vi "Arm Controller.vi"(8 "error in":errorcluster) -> ()   [LabVIEW 2018]
doc: "This VI executes continuously carrying out the current operation and responding to updates or new operations. It will often contain the timing or control code that is difficult to place directly in TeleOp. This VI generally opens all sensors and motors and isolates the rest of the robot code from knowing how the operations are carried out."
uses:
  <vilib>/Rock Robotics/WPI/Framework/Completion Status.ctl
  Arm Setpoints.ctl
  Arm Operations.ctl
  <vilib>/Rock Robotics/SystemInterfaces/AI/FPGA_AIChannel.ctl
  <vilib>/Rock Robotics/WPI/SafetyOutput/WPI_SafetyOutputConfigMenu.ctl
  <vilib>/Rock Robotics/SystemInterfaces/DIO/FPGA_DIOPWMChannel.ctl
  <vilib>/Rock Robotics/WPI/MotorControl/WPI_MotorControlOpen SPARK.vi
panel:
  in  "g":dbl=0.15 format="%#_13g"
  out "POT Angle":dbl
  in  "output range":cluster{"output high":dbl, "output low":dbl}={"output high"=1.0, "output low"=-0.75} {"output low" format="%.2f"; "output high" format="%.2f"}
  in  "PIDF gains":cluster{"Kp":dbl, "Ki":dbl, "Kd":dbl, "Kf":dbl}={"Kp"=0.08, "Ki"=0.0, "Kd"=0.05, "Kf"=0.0} {"Kf" format="%.3f"; "Kd" format="%.3f"; "Ki" format="%.3f"; "Kp" format="%.3f"}
  out "MotorPower":dbl(graph)
  in  "0 voltage":dbl(slide)=2.93 min=0.0 max=5.0 scale=0.0..5.0
  out "POT Voltage":dbl
  out "POT":cluster{"Normalized Value":dbl, "Setpoint":dbl}(graph)
  in  "Max angle":dbl=80.0
  in  "Min angle":dbl=-85.0
  in  "Interactive Values":T1
  out "Current\nCmd":string
  in  "Buttons":cluster{"Execute Cmd":bool, "Abort Cmd":bool}
  out "Command Timing":cluster{"Start Time (ms)":u32, "Iterations":i32}
  out "Status":T3
  # "Interactive Command: You may fill in the settings for a command\nand schedule it with the Execute button. You can observe and abort\nany command while fine tuning the code for the controller."
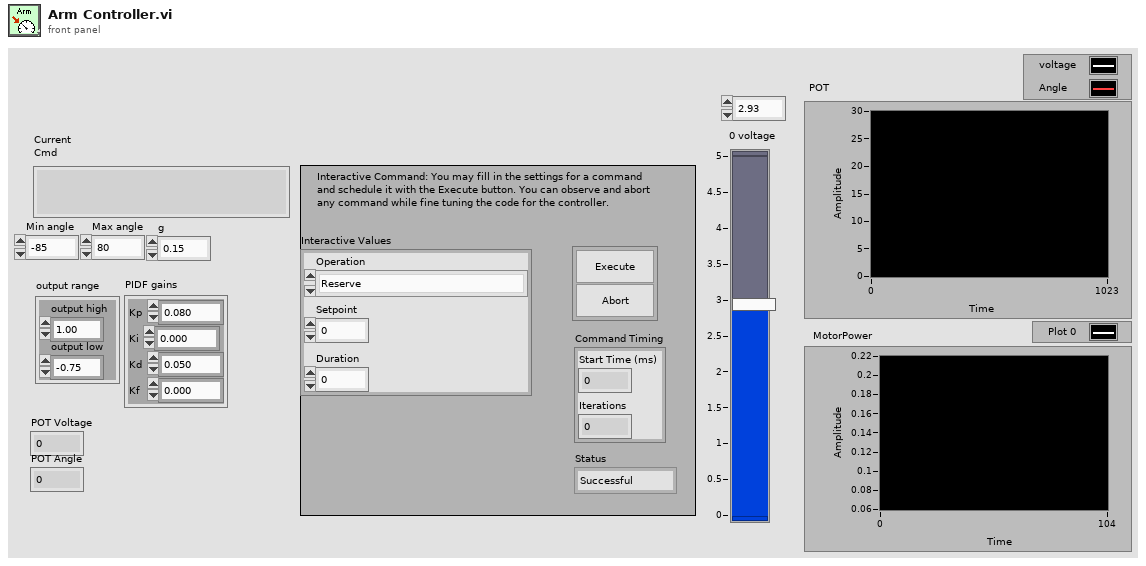
[diagram p1: front panel]
types:
  T1 = typedef "Arm Setpoints.ctl" = cluster{"Operation":T2, "Setpoint":dbl, "Duration":dbl}
  T2 = typedef "Arm Operations.ctl" = enum16{"Reserve", "Read Current", "Turn to angle ", "Set position", "Immediate"}
  T3 = typedef "Completion Status.ctl" = enum16{"Successful", "Aborted", "Incomplete"}
  T4 = typedef "FPGA_DIOPWMChannel.ctl" = enum8{"PWM 0", "PWM 1", "PWM 2", "PWM 3", "PWM 4", "PWM 5", "PWM 6", "PWM 7", "PWM 8", "PWM 9", "PWM MXP 0", "PWM MXP 1", "PWM MXP 2", "PWM MXP 3", "PWM MXP 4", "PWM MXP 5", "PWM MXP 6", "PWM MXP 7", "PWM MXP 8", "PWM MXP 9", "Invalid"}
  T5 = typedef "WPI_SafetyOutputConfigMenu.ctl" = enum16{"Enable", "Disable"}
  T6 = typedef "FPGA_AIChannel.ctl" = enum8{"AI 0", "AI 1", "AI 2", "AI 3", "AI MXP 0", "AI MXP 1", "AI MXP 2", "AI MXP 3", "Invalid"}
  T7 = typedef "WPI_AnalogChannelDevRef.ctl" = cluster{"DevStatus":errorcluster, "Analog Channel":T6}
  T8 = typedef "WPI_MotorControlDeviceRef.ctl" = cluster{"DeviceStatus":errorcluster, "Type":T9, "PWM":cluster{"PWM Channel":T4, "DeadBand":T10}, "CAN":cluster{"Device Number":u8, "SetOutput VI Ref":variant, "GetOutput VI Ref":variant, "Enable VI Ref":variant, "Disable VI Ref":variant, "Data":variant}, "Invert":bool, "DIO PWM":cluster{"PWM \"Enable\" Channel":T4, "DIOChannel":T11, "PWM Rate":dbl}}
  T9 = typedef "WPI_MotorControlType.ctl" = enum16{"PWM", "CAN", "DIO PWM"}
  T10 = typedef "WPI_PWMDeadband.ctl" = cluster{"Name":string, "maxPositivePwm":i32, "minPositivePwm":i32, "centerPwm":i32, "maxNegativePwm":i32, "minNegativePwm":i32, "angularRange":u16}
  T11 = typedef "FPGA_DIOChannel.ctl" = enum8{"DIO 0", "DIO 1", "DIO 2", "DIO 3", "DIO 4", "DIO 5", "DIO 6", "DIO 7", "DIO 8", "DIO 9", "DIO MXP 0", "DIO MXP 1", "DIO MXP 2", "DIO MXP 3", "DIO MXP 4", "DIO MXP 5", "DIO MXP 6", "DIO MXP 7", "DIO MXP 8", "DIO MXP 9", "DIO MXP 10", "DIO MXP 11", "DIO MXP 12", "DIO MXP 13", "DIO MXP 14", "DIO MXP 15", "SPI Port CS1", "SPI Port CS2", "SPI Port CS3", "SPI Port MISO", "SPI Port MOSI", "Invalid"}
  T12 = typedef "Command Status Info.ctl" = cluster{"Name":string, "Status":T3, "notifier out":T13}
  T13 = typedef "Completion Notifier.ctl" = refnum<notifier>
  T14 = cluster{"Current Command":T1, "Command Timing":cluster{"Start Time (ms)":u32, "Iterations":i32}, "Command Arguments":cluster{"Command Info":T12, "Description":string, "Default Command":T1, "queue out":refnum<queue>, "Subsystem Name":string}}
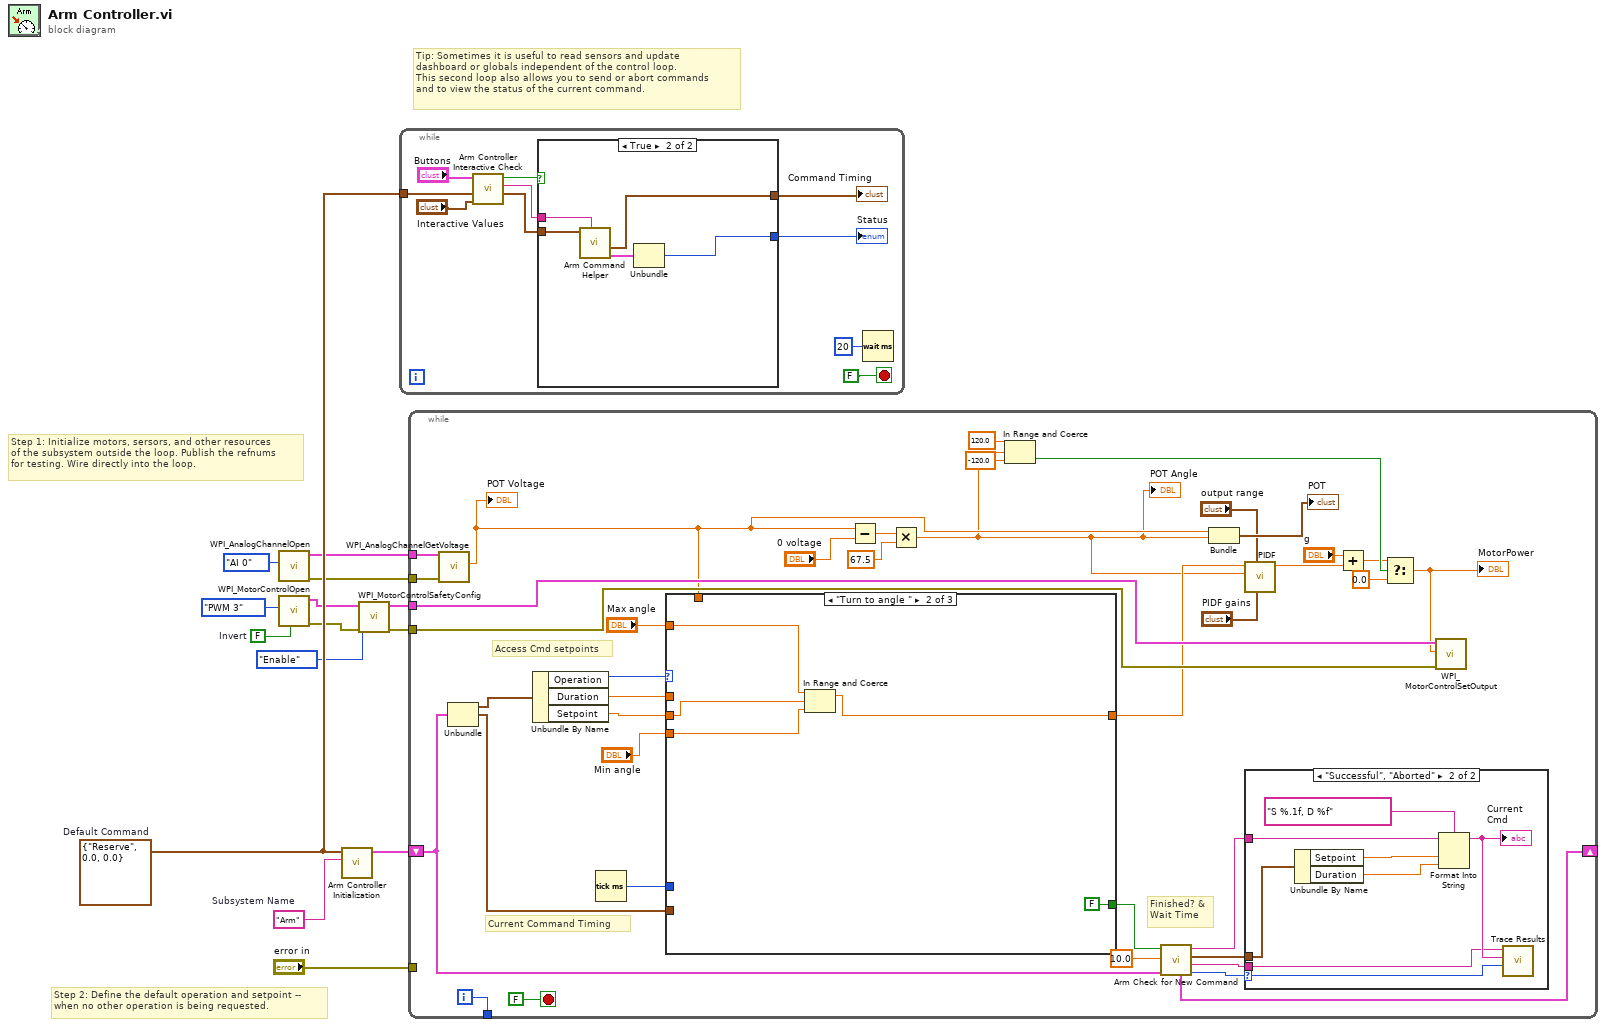
[diagram p0: block diagram]
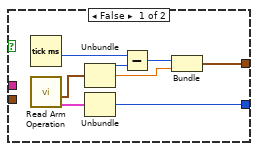
[diagram p2: hidden frame]
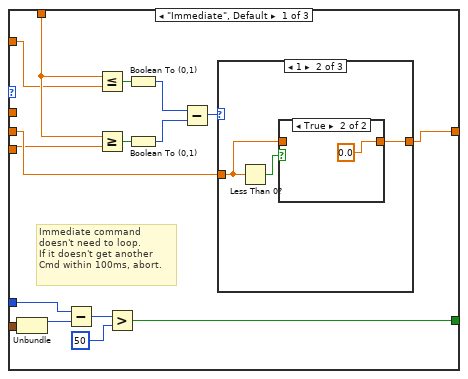
[diagram p4: hidden frame]
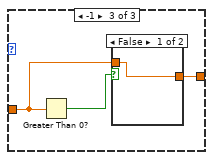
[diagram p7: hidden frame]
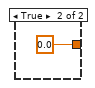
[diagram p8: hidden frame]
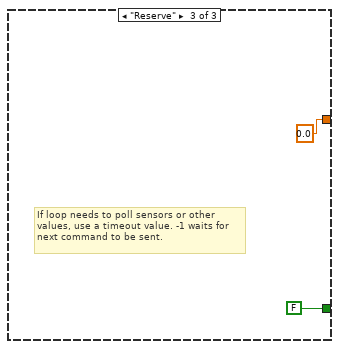
[diagram p9: hidden frame]
diagram:
  w1 = FALSE  # Invert
  w11 = T1 {"Operation"=enum."Reserve", "Setpoint"=0.0, "Duration"=0.0}  # Default Command
  w12 = "Arm"  # Subsystem Name
  # "Tip: Sometimes it is useful to read sensors and update\ndashboard or globals independent of the control loop.\nThis second loop also allows you to send or abort commands\nand to view the status of the current command."
  # "Step 2: Define the default operation and setpoint --\nwhen no other operation is being requested."
  # "Step 1: Initialize motors, sersors, and other resources\nof the subsystem outside the loop. Publish the refnums\nfor testing. Wire directly into the loop."
  n1 = call <vilib>:"WPI_AnalogChannelOpen.vi"("Analog Channel"=FPGA_AIChannel."AI 0") -> ("error out"=w10:errorcluster, "AIDeviceRef"=w9:T7)  [unwired: 9 in]
  n2 = call-poly <vilib>:"WPI_MotorControlOpen.vi"("Invert"=w1, "PWM Channel"=FPGA_DIOPWMChannel."PWM 3") -> ("error out"=w6:errorcluster, "MotorControlDeviceRef"=w7:T8)  [unwired: 8 in]
  n3 = call "Arm Controller Initialization.vi"("Subsystem Name"=w12, "Default Command"=w11) -> ("Current Command"=w13:T14)  [unwired: 9 in]
  n4 = call <vilib>:"WPI_MotorControlSafetyConfig.vi"("error in (no error)"=w6, "mode"=WPI_SafetyOutputConfigMenu."Enable", "MotorControlDevRef"=w7) -> ("error out"=w4:errorcluster, "MotorControlDevRef"=w5:T8)  [unwired: 7 in]
  n5 = while {
    tunnel: w11 -> [w21]
    stop <- FALSE stop-if-true
    n6 = call "Arm Controller Interactive Check.vi"("Interactive Command in"="Interactive Values", "Default Command"=w21, "Buttons"="Buttons") -> ("Interactive Command out"=w18:T1, "Trace String"=w19:string, "Schedule"=w20:bool)  [unwired: 6 in]
    n7 = case shown="True" w20 {
      tunnel: [w32 w37] -> w17
      tunnel: w18 -> [_ w35]
      tunnel: [w28 w33] -> w16
      tunnel: w19 -> [_ w36]
      frame False {
        n8 = Tick Count (ms)() -> (millisecond timer value=w27:u32)
        n9 = call "Read Arm Operation.vi"() -> ("Command Info"=w25:T12, "SubSystem Data"=w26:T1)  [unwired: 9 in, 1 out]
        n10 = Unbundle(w26) -> ("Operation"=w31:T2, "Setpoint"=w29:dbl)  [unwired: 1 out]
        n11 = Unbundle(w25) -> ("Status"=w32:T3)  [unwired: 2 out]
        n12 = Subtract(x=w27, y=w31) -> (x-y=w30:u32)
        n13 = Bundle(w30, "Setpoint"=w29) -> (w28:cluster{u32, "Setpoint":dbl})  [unwired: 1 in]
      }
      frame True {
        n14 = call "Arm Command Helper.vi"("Description"=w36, "SubSystem Data"=w35) -> ("Command Info Out"=w34:T12, "Command Timing"=w33:cluster{"Start Time (ms)":u32, "Iterations":i32})  [unwired: 7 in, 1 out]
        n15 = Unbundle(w34) -> ("Status"=w37:T3)  [unwired: 2 out]
      }
    }
    "Status" <- w17
    "Command Timing" <- w16
    n16 = Wait (ms)(milliseconds to wait=u32 20) -> ()  [unwired: 1 out]
  }
  n17 = while {
    shift-right: [w68] -> _
    shift-left: w13 -> [w62]
    tunnel: [w75] -> _
    tunnel: "error in" -> [_]
    tunnel: w10 -> [w59]
    tunnel: w9 -> [w58]
    tunnel: w5 -> [w56]
    tunnel: w4 -> [w55]
    i -> [w75]
    stop <- FALSE stop-if-true
    # "Current Command Timing"
    # "Access Cmd setpoints"
    # "Finished? &\nWait Time"
    n18 = call <vilib>:"WPI_AnalogChannelGetVoltage.vi"("error in (no error)"=w59, "AIDeviceRef"=w58) -> ("Voltage"=w45:dbl)  [unwired: 7 in, 2 out]
    "POT Voltage" <- w45
    n19 = Unbundle(w62) -> ("Current Command"=w74:T1, "Command Timing"=w70:cluster{"Start Time (ms)":u32, "Iterations":i32})  [unwired: 1 out]
    n20 = Unbundle By Name(w74) -> ("Operation"=w73:T2, "Duration"=w72:dbl, "Setpoint"=w69:dbl)
    n21 = Tick Count (ms)() -> (millisecond timer value=w71:u32)
    n22 = case shown="\"Turn to angle \"" w73 {
      tunnel: [w95 FALSE ("ignore previous (F)") FALSE ("ignore previous (F)")] -> w67
      tunnel: w70 -> [w97 _ _]
      tunnel: w72 -> [_ _ _]
      tunnel: w71 -> [w96 _ _]
      tunnel: w69 -> [w89 w115 _]
      tunnel: "Min angle" -> [w87 w114 _]
      tunnel: "Max angle" -> [w86 w113 _]
      tunnel: w45 -> [w88 _ _]
      tunnel: [w85 w112 0.0 ("Setpoint")] -> w50
      frame "Immediate", Default {
        # "Immediate command\ndoesn't need to loop.\nIf it doesn't get another\nCmd within 100ms, abort."
        n23 = Unbundle(w97) -> ("Start Time (ms)"=w100:u32)  [unwired: 1 out]
        n24 = Subtract(x=w96, y=w100) -> (x-y=w99:u32)
        n25 = Less Or Equal?(x=w88, y=w86) -> (x <= y?=w94:bool)
        n26 = Greater Or Equal?(x=w88, y=w87) -> (x >= y?=w93:bool)
        n27 = Greater?(x=w99, y=u8 50 ("Left Motor")) -> (0:w95:bool)
        n28 = Boolean To (0,1)(Boolean=w94) -> (0, 1=w91:i16)
        n29 = Boolean To (0,1)(Boolean=w93) -> (0, 1=w92:i16)
        n30 = Subtract(x=w91, y=w92) -> (x-y=w90:i16)
        n31 = case shown="1" w90 {
          tunnel: w89 -> [w101 w102 w107]
          tunnel: [w101 w103 w108] -> w85
          frame 0, Default {
          }
          frame 1 {
            n32 = Less Than 0?(x=w102) -> (x < 0?=w104:bool)
            n33 = case shown="True" w104 {
              tunnel: [w105 0.0] -> w103
              tunnel: w102 -> [w105 _]
              frame False {
              }
              frame True {
              }
            }
          }
          frame -1 {
            n34 = Greater Than 0?(x=w107) -> (x > 0?=w109:bool)
            n35 = case shown="False" w109 {
              tunnel: [w110 0.0] -> w108
              tunnel: w107 -> [w110 _]
              frame False {
              }
              frame True {
              }
            }
          }
        }
      }
      frame "Turn to angle " {
        n36 = In Range and Coerce(upper limit=w113, x=w115, lower limit=w114) -> (coerced(x)=w112:dbl)  [unwired: 1 out]
      }
      frame "Reserve" {
        # "If loop needs to poll sensors or other\nvalues, use a timeout value. -1 waits for\nnext command to be sent."
      }
    }
    n37 = Subtract(x=w45, y="0 voltage") -> (x-y=w54:dbl)
    n38 = Multiply(x=w54, y=67.5) -> (x*y=w43:dbl)
    "POT Angle" <- w43
    n39 = In Range and Coerce(upper limit=120.0, x=w43, lower limit=-120.0) -> (In Range?=w40:bool)  [unwired: 1 out]
    n40 = call "Arm Check for New Command.vi"("Current Command"=w62, "Wait time (ms)"=10.0 ("Infinite"), "Finished?"=w67) -> ("Completion"=w63:T3, "Subsystem Name"=w64:string, "Current Command"=w65:T1, "Initial Trace String"=w66:string, "NextCommand"=w68:T14)  [unwired: 4 in]
    n41 = Bundle("Voltage"=w45, w43) -> (→"POT":cluster{"Voltage":dbl, dbl})  [unwired: 1 in]
    n42 = call "PIDF.vi"("PIDF gains"="PIDF gains", "output range"="output range", "process variable"=w43, "setpoint"=w50) -> ("output"=w48:dbl)  [unwired: 5 in, 2 out]
    n43 = case shown="\"Successful\", \"Aborted\"" w63 {
      selector: w63 -> [_ w84]
      tunnel: w66 -> [_ w80]
      tunnel: w65 -> [_ w81]
      tunnel: w64 -> [_ w77]
      frame "Incomplete", Default {
        # "Continuing current command"
      }
      frame "Successful", "Aborted" {
        # "Report and setup for next command"
        n44 = Unbundle By Name(w81) -> ("Setpoint"=w83:dbl, "Duration"=w78:dbl)
        n45 = Format Into String(format string="S %.1f, D %f", initial string=w80, w83, w78) -> (resulting string=w79:string)  [unwired: 1 in, 1 out]
        "Current\nCmd" <- w79
        n46 = call <vilib>:"Trace Results.vi"("Status of previous command"=w84, "Description"=w79, "Subsystem"=w77) -> ()  [unwired: 9 in]
      }
    }
    n47 = Add(x="g", y=w48) -> (x+y=w39:dbl)
    n48 = Select(t=w39, s=w40, f=0.0) -> (s? t:f=w44:dbl)
    "MotorPower" <- w44
    n49 = call <vilib>:"WPI_MotorControlSetOutput.vi"("error in (no error)"=w55, "Output"=w44, "MotorControlDevRef"=w56) -> ()  [unwired: 6 in, 3 out]
  }
